vi "PublishActPos.vi"(4 "AxisNumber":u8, 6 "RawActPos":dbl, 8 "error in (no error)":errorcluster, 11 "CS++Motor in":refnum<class "CS++Motor.lvclass">) -> (0 "error out":errorcluster, 1 "ActPos":dbl, 3 "CS++Motor out":refnum<class "CS++Motor.lvclass">)   [LabVIEW 2015, in "CS++Motor.lvlib" / "CS++Motor.lvclass"]
doc: "This VI publishes the ActPosition."
uses:
  CS++Motor.lvclass
  PV-Enum-n.ctl
  CSPP_Core/Classes/CS++ProcessVariables/ProcessVariable/PV.lvclass
  CS++Motor.lvclass/CS++Motor.ctl
  CSPP_Core/Classes/CS++ProcessVariables/ProcessVariable/PV.lvclass/PV.ctl
  CSPP_Core/Classes/CS++ProcessVariables/ProcessVariable/Write Data.vi
  CSPP_Core/Classes/CS++ProcessVariables/ProcessVariable/Write Timestamp.vi
  CSPP_Core/Classes/CS++ProcessVariables/ProcessVariable/Write Quality.vi
  CSPP_Core/Classes/CS++ProcessVariables/ProcessVariable/Write status.vi
  CSPP_Core/Classes/CS++ProcessVariables/PVConnection/PVConnection.lvclass
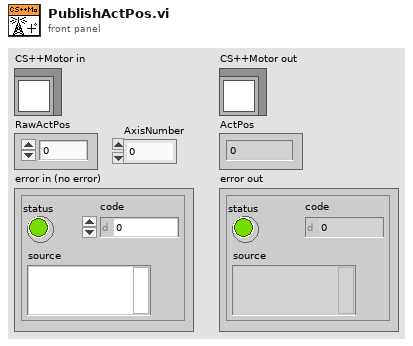
[diagram p1: front panel]
types:
  T1 = typedef "CS++Motor.lvlib/CS++Motor.lvclass/PV-Enum-n.ctl" = enum16{"PhysicalName", "unit", "ActPosition", "SetPosition", "RawSetPosition", "StartVelocity", "StopVelocity", "Acceleration", "RangeMin", "RangeMax", "Scaling", "RangeRefError", "LogicalPositionArray", "NoOfCommands"}
  T2 = cluster{"LogicalName":string, "PhysicalName":string, "unit":string, "Scaling":dbl, "Scaling Offset":dbl, "StartVelocity":dbl, "StopVelocity":dbl, "Acceleration":dbl, "RangeMin":dbl, "RangeMax":dbl, "LogicalPos-Array":cluster{"LogicalPosition":string, "SetPosition":dbl}[]}[]
  T3 = cluster{"LogicalName":string, "PhysicalName":string, "unit":string, "Scaling":dbl, "Scaling Offset":dbl, "StartVelocity":dbl, "StopVelocity":dbl, "Acceleration":dbl, "RangeMin":dbl, "RangeMax":dbl, "LogicalPos-Array":cluster{"LogicalPosition":string, "SetPosition":dbl}[]}
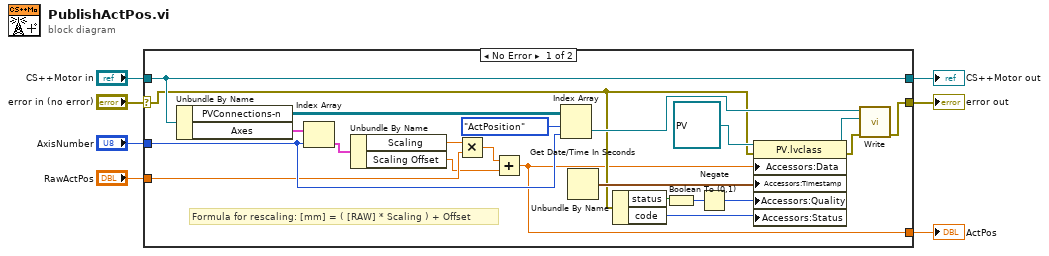
[diagram p0: block diagram]
diagram:
  n1 = case shown="No Error" "error in (no error)" {
    selector: "error in (no error)" -> [w12 w31]
    tunnel: [w11 w31] -> w6
    tunnel: [w27 w30] -> w3
    tunnel: "CS++Motor in" -> [w27 w30]
    tunnel: "RawActPos" -> [w15 _]
    tunnel: "AxisNumber" -> [w24 _]
    tunnel: [w9 _] -> w1
    frame No Error {
      # "Formula for rescaling: [mm] = ( [RAW] * Scaling ) + Offset"
      n2 = Unbundle By Name(w27) -> ("PVConnections-n"=w26:refnum<class "PVConnection.lvclass">[][], "Axes"=w29:T2)
      n3 = Index Array(array=w29, index=w24) -> (element=w28:T3)
      n4 = Unbundle By Name(w28) -> ("Scaling"=w14:dbl, "Scaling Offset"=w8:dbl)
      n5 = Multiply(x=w14, y=w15) -> (x*y=w10:dbl)
      n6 = Add(x=w10, y=w8) -> (x+y=w9:dbl)
      n7 = Index Array(array=w26, index (row)=PV-Enum-n."ActPosition" ("PV-Enum-n"), index (col)=w24) -> (element=w13:refnum<class "PVConnection.lvclass">)
      n8 = Get Date/Time In Seconds() -> (seconds since 1Jan1904=w16:timestamp)
      n9 = Unbundle By Name(w12) -> ("status"=w22:bool, "code"=w19:i32)
      n10 = Boolean To (0,1)(Boolean=w22) -> (0, 1=w18:i16)
      n11 = Negate(x=w18) -> (-x=w23:i16)
      n12 = property class="PV.lvclass"(reference=refnum<class "PV.lvclass"> refnum ("PV"), error in=w12, "Accessors:Data"=w9, "Accessors:Timestamp"=w16, "Accessors:Quality"=w23, "Accessors:Status"=w19) -> (reference out=w21:refnum<class "PV.lvclass">, error out=w20:errorcluster)
      n13 = call "Write.vi"("error in (no error)"=w20, "PV"=w21, "PVConnection in"=w13) -> ("error out"=w11:errorcluster)  [unwired: 7 in, 1 out]
    }
    frame Error {
    }
  }
  "error out" <- w6
  "CS++Motor out" <- w3
  "ActPos" <- w1
